vi "Connection Destroy.vi"(8 "error in (no error)":errorcluster, 11 "Connection DVR in":refnum<data-value>) -> (0 "error out":errorcluster)   [LabVIEW 2015, in "MDSplus.lvlib"]
uses:
  <vilib>/MDSplus/Library/MDSplus.lvlib
  <vilib>/MDSplus/Classes/Connection_Class/Connection.lvclass
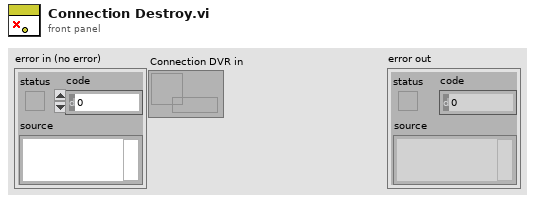
[diagram p1: front panel]
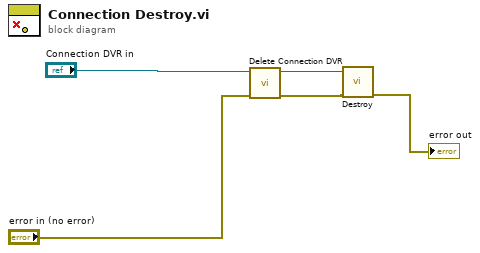
[diagram p0: block diagram]
diagram:
  n1 = call <vilib>:"Delete Connection DVR.vi"("error in (no error)"="error in (no error)", "Connection DVR in"="Connection DVR in") -> ("error out"=w3:errorcluster, "Connection out"=w2:refnum<class "Connection.lvclass">)  [unwired: 8 in]
  n2 = call <vilib>:"Destroy.vi"("error in (no error)"=w3, "Connection in"=w2) -> ("error out"=→"error out":errorcluster)  [unwired: 9 in]
